vi "Identify Calibration Label.vi"(8 "error in":errorcluster, 11 "3022A in":refnum<class "3022A.lvclass">) -> (0 "error out":errorcluster, 2 "Calibration Label":string, 3 "3022A out":refnum<class "3022A.lvclass">)   [LabVIEW 2014, in "3022A.lvclass"]
uses:
  3022A.lvclass
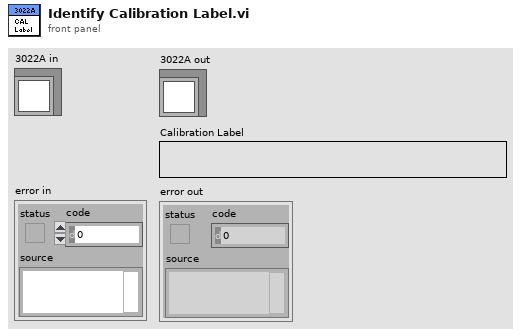
[diagram p1: front panel]
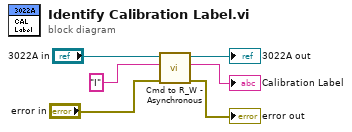
[diagram p0: block diagram]
diagram:
  n1 = call-dynamic "Cmd to R_W - Asynchronous.vi"("error in"="error in", "write buffer"="I", "Serial IO in"="3022A in") -> ("error out"=→"error out":errorcluster, "read buffer"=→"Calibration Label":string, "Serial IO out"=→"3022A out":refnum<class "3022A.lvclass">)  [unwired: 6 in]
